vi "3-1Debugging.vi"() -> ()   [LabVIEW 2024]
panel:
  out "area":dbl
  out "valid is triangle ?":bool
  in  "c":dbl
  in  "b":dbl
  in  "a":dbl
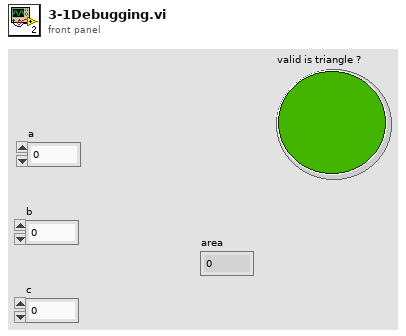
[diagram p1: front panel]
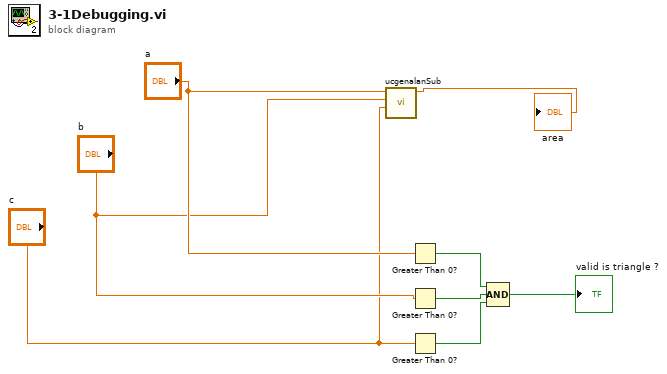
[diagram p0: block diagram]
diagram:
  n1 = call "ucgenalanSub.vi"("Numeric 3"="c", "Numeric 2"="b", "Numeric"="a") -> ("Numeric 4"=→"area":dbl)  [unwired: 8 in]
  n2 = Greater Than 0?(x="a") -> (x > 0?=w6:bool)
  n3 = Greater Than 0?(x="b") -> (x > 0?=w7:bool)
  n4 = Greater Than 0?(x="c") -> (x > 0?=w5:bool)
  n5 = Compound Arithmetic op=AND(w6, w7, w5) -> (→"valid is triangle ?":bool)
